vi "Hex to SGL.vi"(11 "read buffer":string) -> (3 "Data":sgl format="%#_6f")   [LabVIEW 2017]
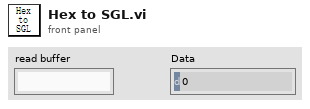
[diagram p1: front panel]
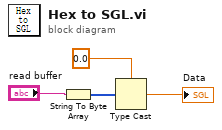
[diagram p0: block diagram]
diagram:
  n1 = String To Byte Array(string="read buffer") -> (unsigned byte array=w2:u8[])
  n2 = Type Cast(type=sgl 0.0, x=w2) -> (*(type *) &x=→"Data":sgl)
